vi "HCC Set Network Variables.vi"(8 "Error In":errorcluster, 11 "Network Var Set":u8=1) -> (0 "Error Out":errorcluster)   [LabVIEW 2016]
uses:
  Utility/Save File/File Setup (Public)/Type Definition/Save File DOE File Path Control.ctl
  Utility/Save File/File Setup (Public)/Type Definition/Save File DOE Data Save Filepaths.ctl
  Utility/Save File/Public/Type Definitions/Save File Washer.ctl
  Utility/Save File/File Setup (Public)/Type Definition/Save File DISH Dishwasher Details.ctl
  <vilib>/Platform/fileVersionInfo.llb/FileVersionInformation.ctl
  Washer DOE/Type Definitions/DOE Appliance Common.ctl
  Utility/Custom Pallet Controls/Custom Pallet String.ctl
  Utility/Save File/File Setup (Public)/Type Definition/DPT IMC Data.ctl
  Washer DOE/Type Definitions/DOE Dryer Standard.ctl
  Utility/Save File/Public/Type Definitions/Save File Appliance Display.ctl
  Utility/Save File/Public/Type Definitions/Save File Unit Type.ctl
  Utility/Save File/Save File.lvlib
  Utility/Save File/File Setup.lvlib
panel:
  # "Set Network Variables"
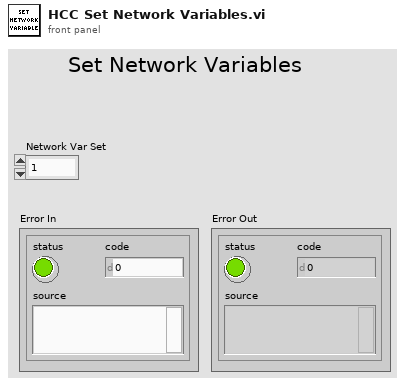
[diagram p1: front panel]
types:
  T1 = typedef "Save File.lvlib/Save File Washer.ctl" = cluster{"Appliance Details":T2, "Display Data (RLT)":T8}
  T2 = typedef "File Setup.lvlib/Save File DISH Dishwasher Details.ctl" = cluster{"FileVersionInfo":T3, "Dishwasher Info":cluster{"Open Cup Weight (gm):":dbl, "Auto Cup Weight (gm):":dbl, "Detergent-Dish:":string, "Inlet Temperature-Dish:":string, "Cycle Mode-Dish:":string, "Unit Control-Dish:":string, "Manufacturer-Dish:":string}, "Washer Info":cluster{"Hot Water Temperature (Fahrenheit):":string, "Cold Water Temperature (Fahrenheit):":string, "Capacity (cu.ft):":dbl, "Initial Cloth Weight:":dbl, "Cloth Lot:":i32, "Model Family:":string, "Program Name:":string, "Cycle Selection:":string, "Wash Temperature:":string, "Rinse Temperature:":string, "Load Size:":string}, "File Name Output Array":string[][], "Calibration Output Array":string[][], "Appliance Common":T4, "Water Heater":cluster{"Heating Mode:":string}, "Dryer":cluster{"Heat Setting:":T5, "Washer Water Temperature (60 ± 5°F):":u16, "Water Hardness (PPM):":u16, "Dryness Setting:":T5, "Dryer Type:":string, "Exhaust:":string, "Drying Cycle:":string, "Load Type:":string, "Nominal Load Weight":string, "Dryer Initial IMC Data":T6}}
  T3 = typedef "FileVersionInformation.ctl" = cluster{"FileVersion":string, "ProductName":string, "InternalName":string, "CompanyName":string, "LegalCopyright":string, "FileDescription":string}
  T4 = typedef "DOE Appliance Common.ctl" = cluster{"Engineer:":string, "Model Number:":string, "Serial Number:":string, "Comments:":string, "Station ID:":string, "Technician:":string, "TR Number:":string, "Lab ID:":string, "Voltage:":string, "Water Pressure (PSI):":string, "Test Date:":string, "Computer Name:":string, "IP Address:":string, "Ambient RH:":string, "Frequency:":string, "Build:":string, "Filename:":string, "Test Type:":string, "Load Run #:":i32, "Ambient Temperature (F):":string, "File Path:":path, "Cycles Per Year":u32}
  T5 = typedef "Custom Pallet String.ctl" = string
  T6 = typedef "DPT IMC Data.ctl" = cluster{"Measured IMC (lbs)":dbl, "Actual Initial RMC (%)":dbl, "RMC (Desired %)":dbl, "Bone Dry Wt(lbs)":dbl, "Tolerance(%)":dbl, "Actual Final RMC (%)":dbl, "CEF (lbf/kWh)":dbl, "Minimum Weight (lbf)":dbl, "Average Weight (lbf)":dbl, "Maximum Weight (lbf)":dbl, "Measured IMC In Range?":bool, "Moisture Reduction Factor":dbl, "Field Use Factor":dbl, "Empty Dryer Cold Weigth":dbl, "Energy Standard":T7, "Weight Cloth (lbs)":dbl, "Relative Moisture Content (%)":dbl, "Relative Moisture Content - Avg (%)":dbl}
  T7 = typedef "DOE Dryer Standard.ctl" = enum16{"D2-Automatic Dryer", "D2-Timer Dryer", "D1-Automatic Dryer", "D1-Timer Dryer", "Other"}
  T8 = typedef "Save File Appliance Display.ctl" = cluster{"Status Color":u32, "Serial Number Display":string, "Cycle Count Display":i32, "Station Label Display":string, "Current Run Start Time Display":dbl, "Board ID Display":string, "RPM Display":u32, "Current Display":dbl, "Current Path Display":path, "Saving Display":bool, "Unit Type Display":T9, "Total Time On Display":dbl, "UI Button":bool}
  T9 = typedef "Save File.lvlib/Save File Unit Type.ctl" = enum32{"", "Viper", "Hawk", "2015"}
  T10 = typedef "File Setup.lvlib/Save File DOE File Path Control.ctl" = cluster{"General Setup Paths":cluster{"Calibration File Path":path, "DOE Capacity Path":path, "Data Folder Path":path, "RLT Backup Data Path":path, "Tool Base Path":path, "General Startup Config Path":path, "File Save Previous Run Path":path, "File Save Configuration Data Path":path}, "Data File Paths":T11, "New Summary Created":bool, "Check Location Interval (Second)":i32}
  T11 = typedef "File Setup.lvlib/Save File DOE Data Save Filepaths.ctl" = cluster{"Data File Path":path, "Debug File Path":path, "Bus Log Path":path, "Current":path, "Summary":path}
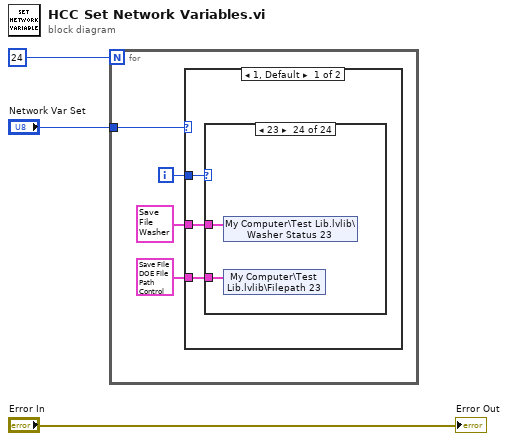
[diagram p0: block diagram]
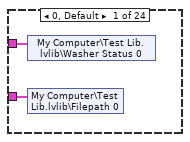
[diagram p2: hidden frame]
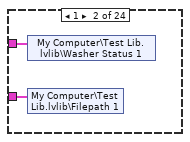
[diagram p3: hidden frame]
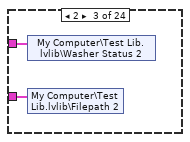
[diagram p4: hidden frame]
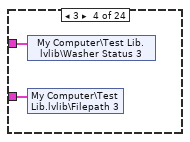
[diagram p5: hidden frame]
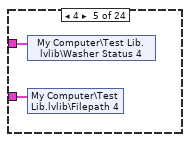
[diagram p6: hidden frame]
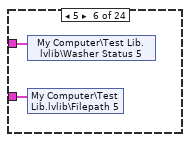
[diagram p7: hidden frame]
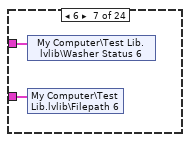
[diagram p8: hidden frame]
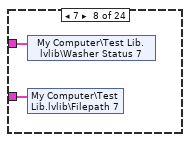
[diagram p9: hidden frame]
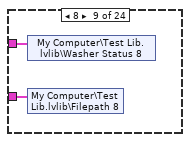
[diagram p10: hidden frame]
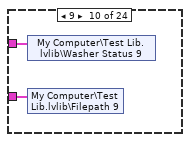
[diagram p11: hidden frame]
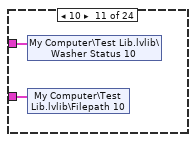
[diagram p12: hidden frame]
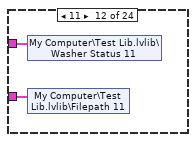
[diagram p13: hidden frame]
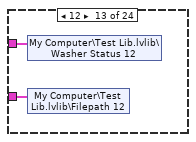
[diagram p14: hidden frame]
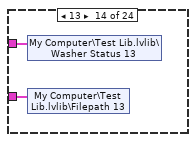
[diagram p15: hidden frame]
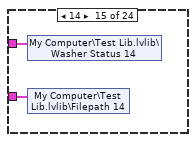
[diagram p16: hidden frame]
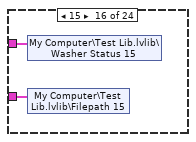
[diagram p17: hidden frame]
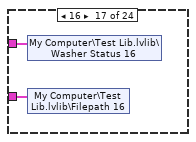
[diagram p18: hidden frame]
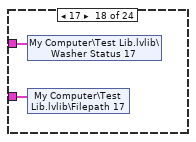
[diagram p19: hidden frame]
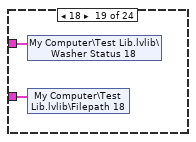
[diagram p20: hidden frame]
diagram:
  n1 = for {
    N: 24 -> [_]
    tunnel: "Network Var Set" -> [w6]
    i -> [w7]
    n2 = case shown="1, Default" w6 {
      tunnel: w7 -> [w10 w61]
      tunnel: T1 {"Appliance Details"={"FileVersionInfo"={"FileVersion"="", "ProductName"="", "InternalName"="", "CompanyName"="", "LegalCopyright"="", "FileDescription"=""}, "Dishwasher Info"={"Open Cup Weight (gm):"=0.0, "Auto Cup Weight (gm):"=0.0, "Detergent-Dish:"="", "Inlet Temperature-Dish:"="", "Cycle Mode-Dish:"="", "Unit Control-Dish:"="", "Manufacturer-Dish:"=""}, "Washer Info"={"Hot Water Temperature (Fahrenheit):"="", "Cold Water Temperature (Fahrenheit):"="", "Capacity (cu.ft):"=0.0, "Initial Cloth Weight:"=0.0, "Cloth Lot:"=0, "Model Family:"="", "Program Name:"="", "Cycle Selection:"="", "Wash Temperature:"="", "Rinse Temperature:"="", "Load Size:"=""}, "File Name Output Array"=[], "Calibration Output Array"=[], "Appliance Common"={"Engineer:"="", "Model Number:"="", "Serial Number:"="", "Comments:"="", "Station ID:"="", "Technician:"="", "TR Number:"="", "Lab ID:"="", "Voltage:"="", "Water Pressure (PSI):"="", "Test Date:"="", "Computer Name:"="", "IP Address:"="", "Ambient RH:"="", "Frequency:"="", "Build:"="", "Filename:"="", "Test Type:"="", "Load Run #:"=0, "Ambient Temperature (F):"="", "File Path:"=path "", "Cycles Per Year"=60}, "Water Heater"={"Heating Mode:"=""}, "Dryer"={"Heat Setting:"="", "Washer Water Temperature (60 ± 5°F):"=60, "Water Hardness (PPM):"=17, "Dryness Setting:"="", "Dryer Type:"="", "Exhaust:"="", "Drying Cycle:"="", "Load Type:"="", "Nominal Load Weight"="", "Dryer Initial IMC Data"={"Measured IMC (lbs)"=7.0, "Actual Initial RMC (%)"=7.0, "RMC (Desired %)"=100.0, "Bone Dry Wt(lbs)"=7.0, "Tolerance(%)"=5.0, "Actual Final RMC (%)"=7.0, "CEF (lbf/kWh)"=0.0, "Minimum Weight (lbf)"=0.0, "Average Weight (lbf)"=0.0, "Maximum Weight (lbf)"=0.0, "Measured IMC In Range?"=FALSE, "Moisture Reduction Factor"=55.5, "Field Use Factor"=1.04, "Empty Dryer Cold Weigth"=0.0, "Energy Standard"=enum."D2-Automatic Dryer", "Weight Cloth (lbs)"=0.0, "Relative Moisture Content (%)"=0.0, "Relative Moisture Content - Avg (%)"=0.0}}}, "Display Data (RLT)"={"Status Color"=0, "Serial Number Display"="", "Cycle Count Display"=0, "Station Label Display"="", "Current Run Start Time Display"=0.0, "Board ID Display"="", "RPM Display"=0, "Current Display"=0.0, "Current Path Display"=path "", "Saving Display"=FALSE, "Unit Type Display"=enum."", "Total Time On Display"=0.0, "UI Button"=FALSE}} ("Dryer") -> [w9 w59]
      tunnel: T10 {"General Setup Paths"={"Calibration File Path"=path "", "DOE Capacity Path"=path "", "Data Folder Path"=path "", "RLT Backup Data Path"=path "", "Tool Base Path"=path "", "General Startup Config Path"=path "", "File Save Previous Run Path"=path "", "File Save Configuration Data Path"=path ""}, "Data File Paths"={"Data File Path"=path "", "Debug File Path"=path "", "Bus Log Path"=path "", "Current"=path "", "Summary"=path ""}, "New Summary Created"=FALSE, "Check Location Interval (Second)"=0} ("Filepath 0") -> [w8 w60]
      frame 1, Default {
        n3 = case shown="23" w10 {
          tunnel: w9 -> [w12 w14 w16 w18 w20 w22 w24 w26 w28 w30 w32 w34 w36 w38 w40 w42 w44 w46 w48 w50 w52 w54 w56 w58]
          tunnel: w8 -> [w11 w13 w15 w17 w19 w21 w23 w25 w27 w29 w31 w33 w35 w37 w39 w41 w43 w45 w47 w49 w51 w53 w55 w57]
          frame 0, Default {
            n4 = shared-variable "My Computer\\Test Lib.lvlib\\Washer Status 0"(w12) -> ()  [unwired: 1 in, 1 out]
            n5 = shared-variable "My Computer\\Test Lib.lvlib\\Filepath 0"(w11) -> ()  [unwired: 1 in, 1 out]
          }
          frame 1 {
            n6 = shared-variable "My Computer\\Test Lib.lvlib\\Washer Status 1"(w14) -> ()  [unwired: 1 in, 1 out]
            n7 = shared-variable "My Computer\\Test Lib.lvlib\\Filepath 1"(w13) -> ()  [unwired: 1 in, 1 out]
          }
          frame 2 {
            n8 = shared-variable "My Computer\\Test Lib.lvlib\\Washer Status 2"(w16) -> ()  [unwired: 1 in, 1 out]
            n9 = shared-variable "My Computer\\Test Lib.lvlib\\Filepath 2"(w15) -> ()  [unwired: 1 in, 1 out]
          }
          frame 3 {
            n10 = shared-variable "My Computer\\Test Lib.lvlib\\Washer Status 3"(w18) -> ()  [unwired: 1 in, 1 out]
            n11 = shared-variable "My Computer\\Test Lib.lvlib\\Filepath 3"(w17) -> ()  [unwired: 1 in, 1 out]
          }
          frame 4 {
            n12 = shared-variable "My Computer\\Test Lib.lvlib\\Washer Status 4"(w20) -> ()  [unwired: 1 in, 1 out]
            n13 = shared-variable "My Computer\\Test Lib.lvlib\\Filepath 4"(w19) -> ()  [unwired: 1 in, 1 out]
          }
          frame 5 {
            n14 = shared-variable "My Computer\\Test Lib.lvlib\\Washer Status 5"(w22) -> ()  [unwired: 1 in, 1 out]
            n15 = shared-variable "My Computer\\Test Lib.lvlib\\Filepath 5"(w21) -> ()  [unwired: 1 in, 1 out]
          }
          frame 6 {
            n16 = shared-variable "My Computer\\Test Lib.lvlib\\Washer Status 6"(w24) -> ()  [unwired: 1 in, 1 out]
            n17 = shared-variable "My Computer\\Test Lib.lvlib\\Filepath 6"(w23) -> ()  [unwired: 1 in, 1 out]
          }
          frame 7 {
            n18 = shared-variable "My Computer\\Test Lib.lvlib\\Washer Status 7"(w26) -> ()  [unwired: 1 in, 1 out]
            n19 = shared-variable "My Computer\\Test Lib.lvlib\\Filepath 7"(w25) -> ()  [unwired: 1 in, 1 out]
          }
          frame 8 {
            n20 = shared-variable "My Computer\\Test Lib.lvlib\\Washer Status 8"(w28) -> ()  [unwired: 1 in, 1 out]
            n21 = shared-variable "My Computer\\Test Lib.lvlib\\Filepath 8"(w27) -> ()  [unwired: 1 in, 1 out]
          }
          frame 9 {
            n22 = shared-variable "My Computer\\Test Lib.lvlib\\Washer Status 9"(w30) -> ()  [unwired: 1 in, 1 out]
            n23 = shared-variable "My Computer\\Test Lib.lvlib\\Filepath 9"(w29) -> ()  [unwired: 1 in, 1 out]
          }
          frame 10 {
            n24 = shared-variable "My Computer\\Test Lib.lvlib\\Washer Status 10"(w32) -> ()  [unwired: 1 in, 1 out]
            n25 = shared-variable "My Computer\\Test Lib.lvlib\\Filepath 10"(w31) -> ()  [unwired: 1 in, 1 out]
          }
          frame 11 {
            n26 = shared-variable "My Computer\\Test Lib.lvlib\\Washer Status 11"(w34) -> ()  [unwired: 1 in, 1 out]
            n27 = shared-variable "My Computer\\Test Lib.lvlib\\Filepath 11"(w33) -> ()  [unwired: 1 in, 1 out]
          }
          frame 12 {
            n28 = shared-variable "My Computer\\Test Lib.lvlib\\Washer Status 12"(w36) -> ()  [unwired: 1 in, 1 out]
            n29 = shared-variable "My Computer\\Test Lib.lvlib\\Filepath 12"(w35) -> ()  [unwired: 1 in, 1 out]
          }
          frame 13 {
            n30 = shared-variable "My Computer\\Test Lib.lvlib\\Washer Status 13"(w38) -> ()  [unwired: 1 in, 1 out]
            n31 = shared-variable "My Computer\\Test Lib.lvlib\\Filepath 13"(w37) -> ()  [unwired: 1 in, 1 out]
          }
          frame 14 {
            n32 = shared-variable "My Computer\\Test Lib.lvlib\\Washer Status 14"(w40) -> ()  [unwired: 1 in, 1 out]
            n33 = shared-variable "My Computer\\Test Lib.lvlib\\Filepath 14"(w39) -> ()  [unwired: 1 in, 1 out]
          }
          frame 15 {
            n34 = shared-variable "My Computer\\Test Lib.lvlib\\Washer Status 15"(w42) -> ()  [unwired: 1 in, 1 out]
            n35 = shared-variable "My Computer\\Test Lib.lvlib\\Filepath 15"(w41) -> ()  [unwired: 1 in, 1 out]
          }
          frame 16 {
            n36 = shared-variable "My Computer\\Test Lib.lvlib\\Washer Status 16"(w44) -> ()  [unwired: 1 in, 1 out]
            n37 = shared-variable "My Computer\\Test Lib.lvlib\\Filepath 16"(w43) -> ()  [unwired: 1 in, 1 out]
          }
          frame 17 {
            n38 = shared-variable "My Computer\\Test Lib.lvlib\\Washer Status 17"(w46) -> ()  [unwired: 1 in, 1 out]
            n39 = shared-variable "My Computer\\Test Lib.lvlib\\Filepath 17"(w45) -> ()  [unwired: 1 in, 1 out]
          }
          frame 18 {
            n40 = shared-variable "My Computer\\Test Lib.lvlib\\Washer Status 18"(w48) -> ()  [unwired: 1 in, 1 out]
            n41 = shared-variable "My Computer\\Test Lib.lvlib\\Filepath 18"(w47) -> ()  [unwired: 1 in, 1 out]
          }
          frame 19 {
            n42 = shared-variable "My Computer\\Test Lib.lvlib\\Washer Status 19"(w50) -> ()  [unwired: 1 in, 1 out]
            n43 = shared-variable "My Computer\\Test Lib.lvlib\\Filepath 19"(w49) -> ()  [unwired: 1 in, 1 out]
          }
          frame 20 {
            n44 = shared-variable "My Computer\\Test Lib.lvlib\\Washer Status 20"(w52) -> ()  [unwired: 1 in, 1 out]
            n45 = shared-variable "My Computer\\Test Lib.lvlib\\Filepath 20"(w51) -> ()  [unwired: 1 in, 1 out]
          }
          frame 21 {
            n46 = shared-variable "My Computer\\Test Lib.lvlib\\Washer Status 21"(w54) -> ()  [unwired: 1 in, 1 out]
            n47 = shared-variable "My Computer\\Test Lib.lvlib\\Filepath 21"(w53) -> ()  [unwired: 1 in, 1 out]
          }
          frame 22 {
            n48 = shared-variable "My Computer\\Test Lib.lvlib\\Washer Status 22"(w56) -> ()  [unwired: 1 in, 1 out]
            n49 = shared-variable "My Computer\\Test Lib.lvlib\\Filepath 22"(w55) -> ()  [unwired: 1 in, 1 out]
          }
          frame 23 {
            n50 = shared-variable "My Computer\\Test Lib.lvlib\\Washer Status 23"(w58) -> ()  [unwired: 1 in, 1 out]
            n51 = shared-variable "My Computer\\Test Lib.lvlib\\Filepath 23"(w57) -> ()  [unwired: 1 in, 1 out]
          }
        }
      }
      frame 2 {
        n52 = case shown="8" w61 {
          tunnel: w59 -> [w62 w64 w66 w68 w70 w72 w74 w76 w78 w80 w82 w84 w86 w88 w90 w92 w94 w96 w98 w100 w102 w104 w106 w108]
          tunnel: w60 -> [w63 w65 w67 w69 w71 w73 w75 w77 w79 w81 w83 w85 w87 w89 w91 w93 w95 w97 w99 w101 w103 w105 w107 w109]
          frame 0, Default {
            n53 = shared-variable "My Computer\\Test Lib.lvlib\\Washer Status 24"(w62) -> ()  [unwired: 1 in, 1 out]
            n54 = shared-variable "My Computer\\Test Lib.lvlib\\Filepath 24"(w63) -> ()  [unwired: 1 in, 1 out]
          }
          frame 1 {
            n55 = shared-variable "My Computer\\Test Lib.lvlib\\Washer Status 25"(w64) -> ()  [unwired: 1 in, 1 out]
            n56 = shared-variable "My Computer\\Test Lib.lvlib\\Filepath 25"(w65) -> ()  [unwired: 1 in, 1 out]
          }
          frame 2 {
            n57 = shared-variable "My Computer\\Test Lib.lvlib\\Washer Status 26"(w66) -> ()  [unwired: 1 in, 1 out]
            n58 = shared-variable "My Computer\\Test Lib.lvlib\\Filepath 26"(w67) -> ()  [unwired: 1 in, 1 out]
          }
          frame 3 {
            n59 = shared-variable "My Computer\\Test Lib.lvlib\\Washer Status 27"(w68) -> ()  [unwired: 1 in, 1 out]
            n60 = shared-variable "My Computer\\Test Lib.lvlib\\Filepath 27"(w69) -> ()  [unwired: 1 in, 1 out]
          }
          frame 4 {
            n61 = shared-variable "My Computer\\Test Lib.lvlib\\Washer Status 28"(w70) -> ()  [unwired: 1 in, 1 out]
            n62 = shared-variable "My Computer\\Test Lib.lvlib\\Filepath 28"(w71) -> ()  [unwired: 1 in, 1 out]
          }
          frame 5 {
            n63 = shared-variable "My Computer\\Test Lib.lvlib\\Washer Status 29"(w72) -> ()  [unwired: 1 in, 1 out]
            n64 = shared-variable "My Computer\\Test Lib.lvlib\\Filepath 29"(w73) -> ()  [unwired: 1 in, 1 out]
          }
          frame 6 {
            n65 = shared-variable "My Computer\\Test Lib.lvlib\\Washer Status 30"(w74) -> ()  [unwired: 1 in, 1 out]
            n66 = shared-variable "My Computer\\Test Lib.lvlib\\Filepath 30"(w75) -> ()  [unwired: 1 in, 1 out]
          }
          frame 7 {
            n67 = shared-variable "My Computer\\Test Lib.lvlib\\Washer Status 31"(w76) -> ()  [unwired: 1 in, 1 out]
            n68 = shared-variable "My Computer\\Test Lib.lvlib\\Filepath 31"(w77) -> ()  [unwired: 1 in, 1 out]
          }
          frame 8 {
            n69 = shared-variable "My Computer\\Test Lib.lvlib\\Washer Status 32"(w78) -> ()  [unwired: 1 in, 1 out]
            n70 = shared-variable "My Computer\\Test Lib.lvlib\\Filepath 32"(w79) -> ()  [unwired: 1 in, 1 out]
          }
          frame 9 {
            n71 = shared-variable "My Computer\\Test Lib.lvlib\\Washer Status 33"(w80) -> ()  [unwired: 1 in, 1 out]
            n72 = shared-variable "My Computer\\Test Lib.lvlib\\Filepath 33"(w81) -> ()  [unwired: 1 in, 1 out]
          }
          frame 10 {
            n73 = shared-variable "My Computer\\Test Lib.lvlib\\Washer Status 34"(w82) -> ()  [unwired: 1 in, 1 out]
            n74 = shared-variable "My Computer\\Test Lib.lvlib\\Filepath 34"(w83) -> ()  [unwired: 1 in, 1 out]
          }
          frame 11 {
            n75 = shared-variable "My Computer\\Test Lib.lvlib\\Washer Status 35"(w84) -> ()  [unwired: 1 in, 1 out]
            n76 = shared-variable "My Computer\\Test Lib.lvlib\\Filepath 35"(w85) -> ()  [unwired: 1 in, 1 out]
          }
          frame 12 {
            n77 = shared-variable "My Computer\\Test Lib.lvlib\\Washer Status 36"(w86) -> ()  [unwired: 1 in, 1 out]
            n78 = shared-variable "My Computer\\Test Lib.lvlib\\Filepath 36"(w87) -> ()  [unwired: 1 in, 1 out]
          }
          frame 13 {
            n79 = shared-variable "My Computer\\Test Lib.lvlib\\Washer Status 37"(w88) -> ()  [unwired: 1 in, 1 out]
            n80 = shared-variable "My Computer\\Test Lib.lvlib\\Filepath 37"(w89) -> ()  [unwired: 1 in, 1 out]
          }
          frame 14 {
            n81 = shared-variable "My Computer\\Test Lib.lvlib\\Washer Status 38"(w90) -> ()  [unwired: 1 in, 1 out]
            n82 = shared-variable "My Computer\\Test Lib.lvlib\\Filepath 38"(w91) -> ()  [unwired: 1 in, 1 out]
          }
          frame 15 {
            n83 = shared-variable "My Computer\\Test Lib.lvlib\\Washer Status 39"(w92) -> ()  [unwired: 1 in, 1 out]
            n84 = shared-variable "My Computer\\Test Lib.lvlib\\Filepath 39"(w93) -> ()  [unwired: 1 in, 1 out]
          }
          frame 16 {
            n85 = shared-variable "My Computer\\Test Lib.lvlib\\Washer Status 40"(w94) -> ()  [unwired: 1 in, 1 out]
            n86 = shared-variable "My Computer\\Test Lib.lvlib\\Filepath 40"(w95) -> ()  [unwired: 1 in, 1 out]
          }
          frame 17 {
            n87 = shared-variable "My Computer\\Test Lib.lvlib\\Washer Status 41"(w96) -> ()  [unwired: 1 in, 1 out]
            n88 = shared-variable "My Computer\\Test Lib.lvlib\\Filepath 41"(w97) -> ()  [unwired: 1 in, 1 out]
          }
          frame 18 {
            n89 = shared-variable "My Computer\\Test Lib.lvlib\\Washer Status 42"(w98) -> ()  [unwired: 1 in, 1 out]
            n90 = shared-variable "My Computer\\Test Lib.lvlib\\Filepath 42"(w99) -> ()  [unwired: 1 in, 1 out]
          }
          frame 19 {
            n91 = shared-variable "My Computer\\Test Lib.lvlib\\Washer Status 43"(w100) -> ()  [unwired: 1 in, 1 out]
            n92 = shared-variable "My Computer\\Test Lib.lvlib\\Filepath 43"(w101) -> ()  [unwired: 1 in, 1 out]
          }
          frame 20 {
            n93 = shared-variable "My Computer\\Test Lib.lvlib\\Washer Status 44"(w102) -> ()  [unwired: 1 in, 1 out]
            n94 = shared-variable "My Computer\\Test Lib.lvlib\\Filepath 44"(w103) -> ()  [unwired: 1 in, 1 out]
          }
          frame 21 {
            n95 = shared-variable "My Computer\\Test Lib.lvlib\\Washer Status 45"(w104) -> ()  [unwired: 1 in, 1 out]
            n96 = shared-variable "My Computer\\Test Lib.lvlib\\Filepath 45"(w105) -> ()  [unwired: 1 in, 1 out]
          }
          frame 22 {
            n97 = shared-variable "My Computer\\Test Lib.lvlib\\Washer Status 46"(w106) -> ()  [unwired: 1 in, 1 out]
            n98 = shared-variable "My Computer\\Test Lib.lvlib\\Filepath 46"(w107) -> ()  [unwired: 1 in, 1 out]
          }
          frame 23 {
            n99 = shared-variable "My Computer\\Test Lib.lvlib\\Washer Status 47"(w108) -> ()  [unwired: 1 in, 1 out]
            n100 = shared-variable "My Computer\\Test Lib.lvlib\\Filepath 47"(w109) -> ()  [unwired: 1 in, 1 out]
          }
        }
      }
    }
  }
  "Error Out" <- "Error In"
